vi "enqueueTelToClient.vi"(8 "error in (no error)":errorcluster, 9 "queueOptions":T1={"EnqueueOptions"=enum."normal enqueue", "Timeout"=0}, 10 "elements to enqueue":string, 11 "TcpServerTel in":refnum<class "TcpServerTel.lvclass">) -> (0 "error out":errorcluster, 3 "TcpServerTel out":refnum<class "TcpServerTel.lvclass">)   [LabVIEW 2018, in "TcpServerTel.lvclass"]
doc: "Enqueue elements into queueTel through Lossy Enqueue Element or Enqueue Element functions. Use lossy enqueue option to implement a circular buffer and un-block call technique. Use normal enqueue option to implement block/un-block call using the timeout value."
uses:
  TcpServerTel.lvclass
  typedef/queueOptionsTypeDef.ctl
  typedef/enqueueOptionsTypeDef.ctl
  home/pcortes/github/ts_labview_tcp_json/src/TcpServerBase/TcpServerBase.lvclass
  TcpServerBase/TcpServerBase.lvclass/TcpServerBase.ctl
  TcpServerBase/TcpServerBase.lvclass
panel:
  out "tcpClientQueueOverflow":bool
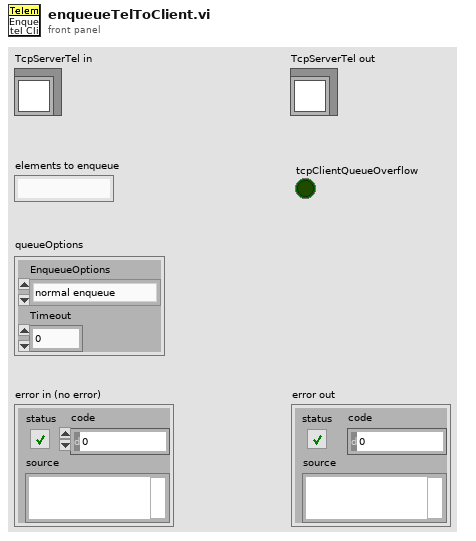
[diagram p1: front panel]
types:
  T1 = typedef "TcpServerTel.lvclass/queueOptionsTypeDef.ctl" = cluster{"EnqueueOptions":T2, "Timeout":i32}
  T2 = typedef "TcpServerTel.lvclass/enqueueOptionsTypeDef.ctl" = enum16{"lossy enqueue", "normal enqueue"}
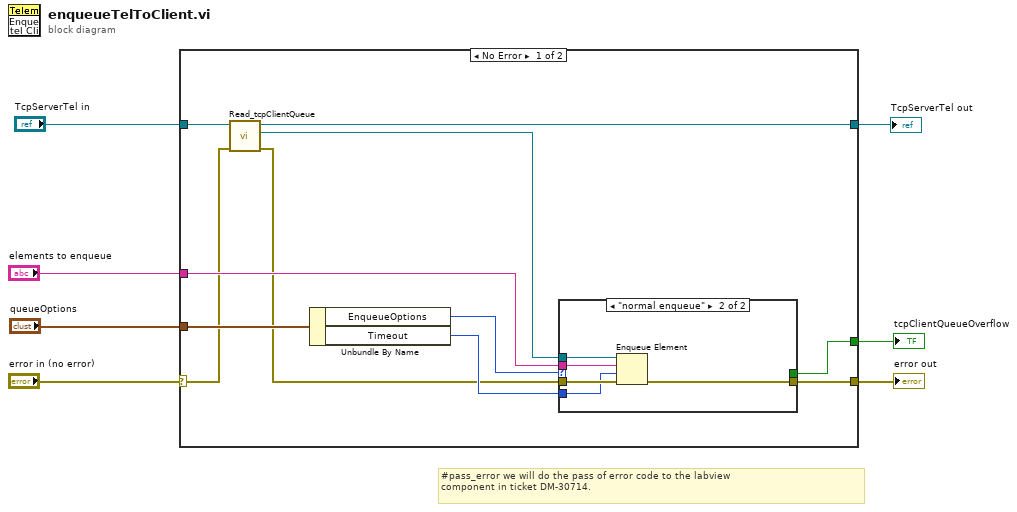
[diagram p0: block diagram]
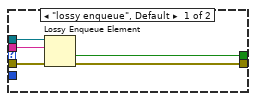
[diagram p2: hidden frame]
diagram:
  # "#pass_error we will do the pass of error code to the labview \ncomponent in ticket DM-30714."
  n1 = case shown="No Error" "error in (no error)" {
    selector: "error in (no error)" -> [w9 w29]
    tunnel: [w18 w29] -> w7
    tunnel: "elements to enqueue" -> [w17 _]
    tunnel: [w16 _] -> w5
    tunnel: "queueOptions" -> [w15 _]
    tunnel: "TcpServerTel in" -> [w14 w30]
    tunnel: [w10 w30] -> w2
    frame No Error {
      n2 = call "Read_tcpClientQueue.vi"("error in (no error)"=w9, "TcpServerBase in"=w14) -> ("error out"=w8:errorcluster, "tcpClientQueue"=w11:refnum<queue>, "TcpServerBase out"=w10:refnum<class "TcpServerTel.lvclass">)  [unwired: 7 in]
      n3 = Unbundle By Name(w15) -> ("EnqueueOptions"=w13:T2, "Timeout"=w12:i32)
      n4 = case shown="\"normal enqueue\"" w13 {
        tunnel: [w23 w27] -> w18
        tunnel: w8 -> [w22 w28]
        tunnel: w17 -> [w21 w25]
        tunnel: w11 -> [w20 w26]
        tunnel: [w19 _] -> w16
        tunnel: w12 -> [_ w24]
        frame "lossy enqueue", Default {
          n5 = Lossy Enqueue Element(queue=w20, element=w21, error in (no error)=w22) -> (overflow?=w19:bool, error out=w23:errorcluster)  [unwired: 2 out]
        }
        frame "normal enqueue" {
          n6 = Enqueue Element(queue=w26, element=w25, timeout in ms (-1)=w24, error in (no error)=w28) -> (error out=w27:errorcluster)  [unwired: 2 out]
        }
      }
    }
    frame Error {
    }
  }
  "error out" <- w7
  "tcpClientQueueOverflow" <- w5
  "TcpServerTel out" <- w2
